vi "Left Initialization (SubVI).vi"   [LabVIEW 2015]
uses:
  Left Variables.vi
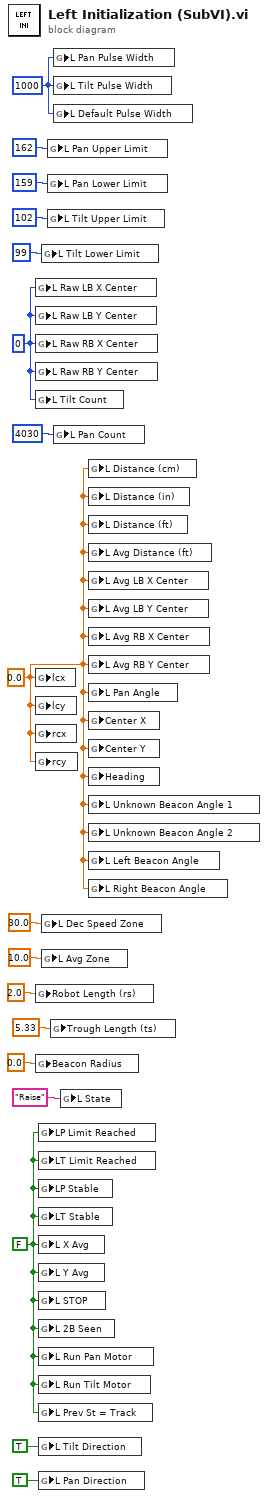
[diagram p0: block diagram]
diagram:
  w2 = u32 1000 ("Pan Upper Limit")
  w4 = u16 0 ("L Raw LB X Center")
  w1 = FALSE ("L Limit Reached")
  w3 = 0.0 ("R Distance (cm)")
  n1 = global write "Left Variables.vi" "L Raw LB X Center"(w4) -> ()
  n2 = global write "Left Variables.vi" "L Raw LB Y Center"(w4) -> ()
  n3 = global write "Left Variables.vi" "L Raw RB X Center"(w4) -> ()
  n4 = global write "Left Variables.vi" "L Raw RB Y Center"(w4) -> ()
  n5 = global write "Left Variables.vi" "L Tilt Count"(w4) -> ()
  n6 = global write "Left Variables.vi" "lcx"(w3) -> ()
  n7 = global write "Left Variables.vi" "lcy"(w3) -> ()
  n8 = global write "Left Variables.vi" "rcx"(w3) -> ()
  n9 = global write "Left Variables.vi" "rcy"(w3) -> ()
  n10 = global write "Left Variables.vi" "Robot Length (rs)"(2.0 ("Dead Zone")) -> ()
  n11 = global write "Left Variables.vi" "Beacon Radius"(0.0 ("Dead Zone")) -> ()
  n12 = global write "Left Variables.vi" "LP Limit Reached"(w1) -> ()
  n13 = global write "Left Variables.vi" "LT Limit Reached"(w1) -> ()
  n14 = global write "Left Variables.vi" "LP Stable"(w1) -> ()
  n15 = global write "Left Variables.vi" "LT Stable"(w1) -> ()
  n16 = global write "Left Variables.vi" "L X Avg"(w1) -> ()
  n17 = global write "Left Variables.vi" "L Y Avg"(w1) -> ()
  n18 = global write "Left Variables.vi" "L STOP"(w1) -> ()
  n19 = global write "Left Variables.vi" "L 2B Seen"(w1) -> ()
  n20 = global write "Left Variables.vi" "L Run Pan Motor"(w1) -> ()
  n21 = global write "Left Variables.vi" "L Run Tilt Motor"(w1) -> ()
  n22 = global write "Left Variables.vi" "L Prev St = Track"(w1) -> ()
  n23 = global write "Left Variables.vi" "L Tilt Direction"(TRUE ("L Tilt Direction")) -> ()
  n24 = global write "Left Variables.vi" "L Pan Direction"(TRUE ("L Pan Direction")) -> ()
  n25 = global write "Left Variables.vi" "L Tilt Lower Limit"(u16 99 ("Tilt Lower Limit")) -> ()
  n26 = global write "Left Variables.vi" "L Dec Speed Zone"(30.0 ("Dead Zone")) -> ()
  n27 = global write "Left Variables.vi" "L Avg Zone"(10.0 ("Dead Zone")) -> ()
  n28 = global write "Left Variables.vi" "L Pan Upper Limit"(u16 162 ("Pan Upper Limit")) -> ()
  n29 = global write "Left Variables.vi" "L Pan Lower Limit"(u16 159 ("Pan Lower Limit")) -> ()
  n30 = global write "Left Variables.vi" "L Tilt Upper Limit"(u16 102 ("Tilt Upper Limit")) -> ()
  n31 = global write "Left Variables.vi" "Trough Length (ts)"(5.33 ("Dead Zone")) -> ()
  n32 = global write "Left Variables.vi" "L Pan Pulse Width"(w2) -> ()
  n33 = global write "Left Variables.vi" "L Tilt Pulse Width"(w2) -> ()
  n34 = global write "Left Variables.vi" "L Default Pulse Width"(w2) -> ()
  n35 = global write "Left Variables.vi" "L Pan Count"(4030 ("L Pan Count")) -> ()
  n36 = global write "Left Variables.vi" "L State"("Raise" ("R State")) -> ()
  n37 = global write "Left Variables.vi" "L Distance (cm)"(w3) -> ()
  n38 = global write "Left Variables.vi" "L Distance (in)"(w3) -> ()
  n39 = global write "Left Variables.vi" "L Distance (ft)"(w3) -> ()
  n40 = global write "Left Variables.vi" "L Avg Distance (ft)"(w3) -> ()
  n41 = global write "Left Variables.vi" "L Avg LB X Center"(w3) -> ()
  n42 = global write "Left Variables.vi" "L Avg LB Y Center"(w3) -> ()
  n43 = global write "Left Variables.vi" "L Avg RB X Center"(w3) -> ()
  n44 = global write "Left Variables.vi" "L Avg RB Y Center"(w3) -> ()
  n45 = global write "Left Variables.vi" "L Pan Angle"(w3) -> ()
  n46 = global write "Left Variables.vi" "Center X"(w3) -> ()
  n47 = global write "Left Variables.vi" "Center Y"(w3) -> ()
  n48 = global write "Left Variables.vi" "Heading"(w3) -> ()
  n49 = global write "Left Variables.vi" "L Unknown Beacon Angle 1"(w3) -> ()
  n50 = global write "Left Variables.vi" "L Unknown Beacon Angle 2"(w3) -> ()
  n51 = global write "Left Variables.vi" "L Left Beacon Angle"(w3) -> ()
  n52 = global write "Left Variables.vi" "L Right Beacon Angle"(w3) -> ()
